vi "Header Names TWIN.vi"(11 "Dynamic Data":dynamicdata(waveform)) -> (3 "Signals Out":dynamicdata(waveform))   [LabVIEW 2017]
uses:
  <vilib>/express/express shared/transition.llb/Dynamic To Waveform Array.vi
  <vilib>/express/express signal manip/GetorSetDDTAttributes/Set DDT Attributes/SetT0.vi
  <vilib>/express/express shared/transition.llb/Waveform Array To Dynamic.vi
  <vilib>/express/express signal manip/GetorSetDDTAttributes/Set DDT Attributes/Set DDT Properties.xnode
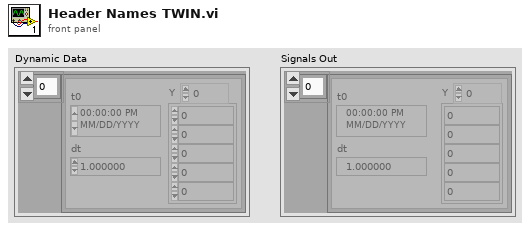
[diagram p1: front panel]
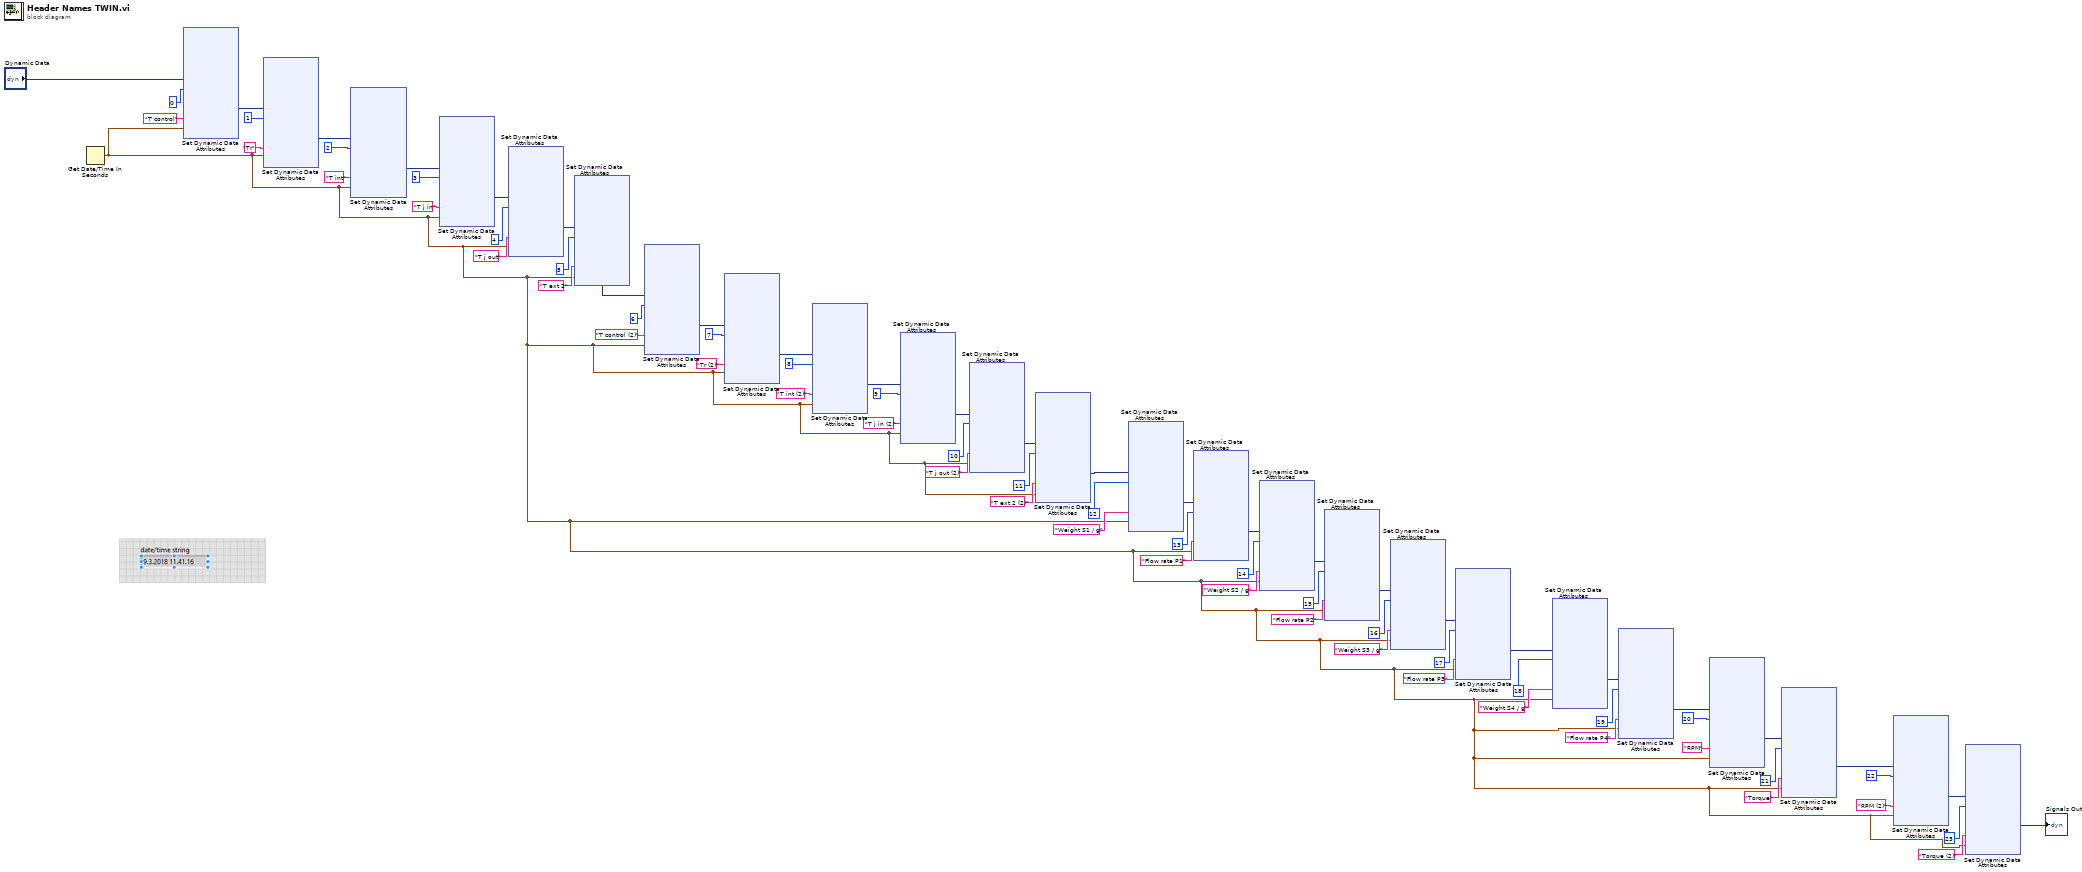
[diagram p0: block diagram]
diagram:
  n1 = Get Date/Time In Seconds() -> (seconds since 1Jan1904=w2:timestamp)
  n2 = xnode "Set Dynamic Data Attributes"("Signals In"="Dynamic Data", "Signal Index"=0, "Signal Name"="T control", "Timestamp"=w2) -> ("Signals Out"=w42:dynamicdata)  [unwired: 1 in, 1 out]
  n3 = xnode "Set Dynamic Data Attributes"("Signals In"=w42, "Signal Index"=1, "Signal Name"="Tr", "Timestamp"=w2) -> ("Signals Out"=w43:dynamicdata)  [unwired: 1 in, 1 out]
  n4 = xnode "Set Dynamic Data Attributes"("Signals In"=w43, "Signal Index"=2, "Signal Name"="T int", "Timestamp"=w2) -> ("Signals Out"=w46:dynamicdata)  [unwired: 1 in, 1 out]
  n5 = xnode "Set Dynamic Data Attributes"("Signals In"=w46, "Signal Index"=3, "Signal Name"="T j in", "Timestamp"=w2) -> ("Signals Out"=w49:dynamicdata)  [unwired: 1 in, 1 out]
  n6 = xnode "Set Dynamic Data Attributes"("Signals In"=w49, "Signal Index"=4, "Signal Name"="T j out", "Timestamp"=w2) -> ("Signals Out"=w52:dynamicdata)  [unwired: 1 in, 1 out]
  n7 = xnode "Set Dynamic Data Attributes"("Signals In"=w52, "Signal Index"=5, "Signal Name"="T ext 2", "Timestamp"=w2) -> ("Signals Out"=w17:dynamicdata)  [unwired: 1 in, 1 out]
  n8 = xnode "Set Dynamic Data Attributes"("Signals In"=w17, "Signal Index"=6, "Signal Name"="T control (2)", "Timestamp"=w2) -> ("Signals Out"=w24:dynamicdata)  [unwired: 1 in, 1 out]
  n9 = xnode "Set Dynamic Data Attributes"("Signals In"=w24, "Signal Index"=7, "Signal Name"="Tr (2)", "Timestamp"=w2) -> ("Signals Out"=w25:dynamicdata)  [unwired: 1 in, 1 out]
  n10 = xnode "Set Dynamic Data Attributes"("Signals In"=w25, "Signal Index"=8, "Signal Name"="T int (2)", "Timestamp"=w2) -> ("Signals Out"=w28:dynamicdata)  [unwired: 1 in, 1 out]
  n11 = xnode "Set Dynamic Data Attributes"("Signals In"=w28, "Signal Index"=9, "Signal Name"="T j in (2)", "Timestamp"=w2) -> ("Signals Out"=w31:dynamicdata)  [unwired: 1 in, 1 out]
  n12 = xnode "Set Dynamic Data Attributes"("Signals In"=w31, "Signal Index"=10, "Signal Name"="T j out (2)", "Timestamp"=w2) -> ("Signals Out"=w34:dynamicdata)  [unwired: 1 in, 1 out]
  n13 = xnode "Set Dynamic Data Attributes"("Signals In"=w34, "Signal Index"=11, "Signal Name"="T ext 2 (2)", "Timestamp"=w2) -> ("Signals Out"=w16:dynamicdata)  [unwired: 1 in, 1 out]
  n14 = xnode "Set Dynamic Data Attributes"("Signals In"=w16, "Signal Index"=12, "Signal Name"="Weight S1 / g", "Timestamp"=w2) -> ("Signals Out"=w59:dynamicdata)  [unwired: 1 in, 1 out]
  n15 = xnode "Set Dynamic Data Attributes"("Signals In"=w59, "Signal Index"=13, "Signal Name"="Flow rate P1", "Timestamp"=w2) -> ("Signals Out"=w60:dynamicdata)  [unwired: 1 in, 1 out]
  n16 = xnode "Set Dynamic Data Attributes"("Signals In"=w60, "Signal Index"=14, "Signal Name"="Weight S2 / g", "Timestamp"=w2) -> ("Signals Out"=w63:dynamicdata)  [unwired: 1 in, 1 out]
  n17 = xnode "Set Dynamic Data Attributes"("Signals In"=w63, "Signal Index"=15, "Signal Name"="Flow rate P2", "Timestamp"=w2) -> ("Signals Out"=w66:dynamicdata)  [unwired: 1 in, 1 out]
  n18 = xnode "Set Dynamic Data Attributes"("Signals In"=w66, "Signal Index"=16, "Signal Name"="Weight S3 / g", "Timestamp"=w2) -> ("Signals Out"=w69:dynamicdata)  [unwired: 1 in, 1 out]
  n19 = xnode "Set Dynamic Data Attributes"("Signals In"=w69, "Signal Index"=17, "Signal Name"="Flow rate P3", "Timestamp"=w2) -> ("Signals Out"=w10:dynamicdata)  [unwired: 1 in, 1 out]
  n20 = xnode "Set Dynamic Data Attributes"("Signals In"=w10, "Signal Index"=18, "Signal Name"="Weight S4 / g", "Timestamp"=w2) -> ("Signals Out"=w15:dynamicdata)  [unwired: 1 in, 1 out]
  n21 = xnode "Set Dynamic Data Attributes"("Signals In"=w15, "Signal Index"=19, "Signal Name"="Flow rate P4", "Timestamp"=w2) -> ("Signals Out"=w9:dynamicdata)  [unwired: 1 in, 1 out]
  n22 = xnode "Set Dynamic Data Attributes"("Signals In"=w9, "Signal Index"=20, "Signal Name"="RPM", "Timestamp"=w2) -> ("Signals Out"=w74:dynamicdata)  [unwired: 1 in, 1 out]
  n23 = xnode "Set Dynamic Data Attributes"("Signals In"=w74, "Signal Index"=21, "Signal Name"="Torque", "Timestamp"=w2) -> ("Signals Out"=w3:dynamicdata)  [unwired: 1 in, 1 out]
  n24 = xnode "Set Dynamic Data Attributes"("Signals In"=w3, "Signal Index"=22, "Signal Name"="RPM (2)", "Timestamp"=w2) -> ("Signals Out"=w8:dynamicdata)  [unwired: 1 in, 1 out]
  n25 = xnode "Set Dynamic Data Attributes"("Signals In"=w8, "Signal Index"=23, "Signal Name"="Torque (2)", "Timestamp"=w2) -> ("Signals Out"=→"Signals Out":dynamicdata)  [unwired: 1 in, 1 out]
